vi "Read Display Bar Graph Configuration.vi"(8 "error in (no error)":errorcluster, 11 "VGC in":refnum<class "PL Inficon VGC.lvclass">) -> (0 "error out":errorcluster, 1 "graph mode":u16(ring) items=["off", "full scale", "full scale, high level", "full scale, setpoint", "decade", "decade, high level", "decade setpoint", "f(t), 0.2 s/pixel", "f(t), 1 s/pixel", "f(t), 6 s/pixel", "f(t), 1 min./pixel"], 2 "channel":u16(ring) items=["channel 1", "channel 2", "channel 3"], 3 "VGC out":refnum<class "PL Inficon VGC.lvclass">)   [LabVIEW 2015, in "PL Inficon VGC.lvclass"]
doc: "Reads display bar graph configuration."
uses:
  PL Inficon VGC.lvclass
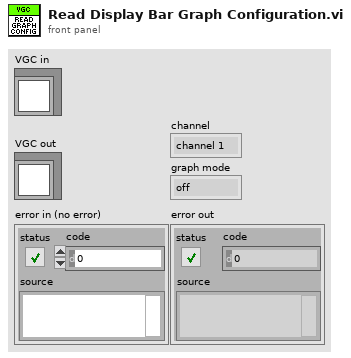
[diagram p1: front panel]
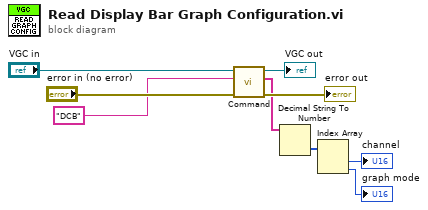
[diagram p0: block diagram]
diagram:
  n1 = call "Command.vi"("error in (no error)"="error in (no error)", "command"="DCB" ("format string"), "VGC in"="VGC in") -> ("error out"=→"error out":errorcluster, "response data"=w4:string[], "VGC out"=→"VGC out":refnum<class "PL Inficon VGC.lvclass">)  [unwired: 6 in]
  n2 = Decimal String To Number(string=w4) -> (number=w5:i32[])  [unwired: 2 in, 1 out]
  n3 = Index Array(array=w5) -> (element #1=→"channel":i32, element #2=→"graph mode":i32)  [unwired: 2 in]
